vi "Do.vi"(8 "error in (no error)":errorcluster, 10 "Actor in":refnum<class "Actor.lvclass">, 11 "Insert Bound View Msg":refnum<class "Insert Bound View Msg.lvclass">) -> (0 "error out":errorcluster, 2 "Actor out":refnum<class "Actor.lvclass">)   [LabVIEW 2019, in "BoundViewManager.lvlib" / "Insert Bound View Msg.lvclass"]
doc: "(<B>Filename</B>: Actor Framework.lvlib:Message.lvclass:Do.vi)\n\nDefines what a message does when it is received by an actor. Generally, a message instructs an actor to invoke one of its methods. By default, this method does nothing. A child class must override it to define behavior. Create a child class by using the Actor Framework Message Maker dialog box."
uses:
  <vilib>/gpm_packages/@cs/ViewManager/source/BoundViewManager Messages/Insert Bound View Msg/Insert Bound View Msg.lvclass
  <vilib>/ActorFramework/Actor/Actor.lvclass
  <vilib>/gpm_packages/@cs/ViewManager/source/BoundViewManager/BoundViewManager.lvclass
  C:/Program Files/National Instruments/LabVIEW 2019/vi.lib/ActorFramework/Actor/Actor.lvclass
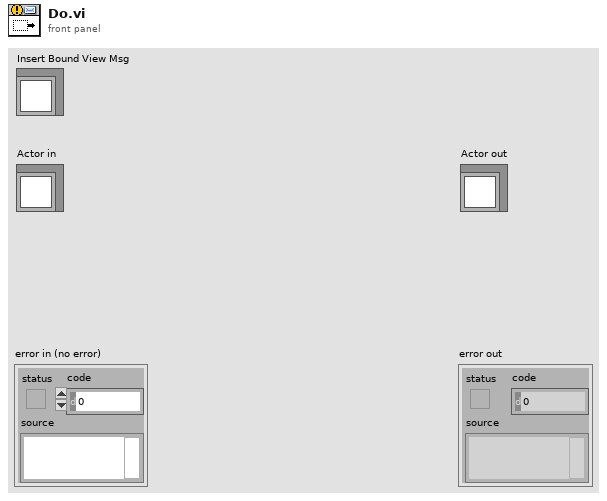
[diagram p1: front panel]
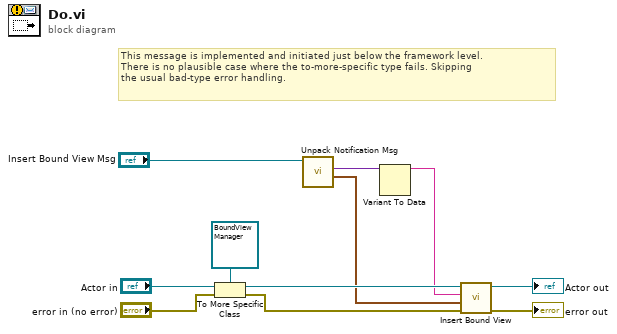
[diagram p0: block diagram]
diagram:
  # "This message is implemented and initiated just below the framework level.\nThere is no plausible case where the to-more-specific type fails. Skipping\nthe usual bad-type error handling."
  n1 = To More Specific Class(target class=refnum<class "BoundViewManager.lvclass"> refnum ("BoundViewManager.lvlib:BoundViewManager.lvclass"), reference="Actor in", error in="error in (no error)") -> (specific class reference=w9:refnum<class "BoundViewManager.lvclass">, error out=w7:errorcluster)
  n2 = call-dynamic "Unpack Notification Msg.vi"("Notification Msg"="Insert Bound View Msg") -> ("Publication Time"=w5:timestamp, "Value"=w4:variant)  [unwired: 8 in, 1 out]
  n3 = Variant To Data(Variant=w4) -> (data=w3:string)  [unwired: 2 in, 1 out]
  n4 = call-dynamic "Insert Bound View.vi"("error in (no error)"=w7, "Value Publication Time"=w5, "Selector Value"=w3, "BoundViewManager in"=w9) -> ("error out"=→"error out":errorcluster, "BoundViewManager out"=→"Actor out":refnum<class "BoundViewManager.lvclass">)  [unwired: 6 in]
